vi "ColorPatternMatch_Setting_UI.vi"(0 "Vision_Image In":T3(plugin-control), 1 "Coord?":bool, 5 "List ROI 2":refnum<vi>, 7 "AlgIn":T2, 9 "ProjectName":string="CDF", 11 "error in (no error)":errorcluster, 12 "Parameter":string, 14 "RootPath":path) -> (4 "Analysis_Setting":string, 10 "Cancel?":bool, 15 "error out":errorcluster)   [LabVIEW 2019]
uses:
  Controls/V_Analysis_Type.ctl
  Controls/_UI Command Cluster/ColorMatch_UI Command.ctl
  <vilib>/Utility/miscctls.llb/LVPointTypeDef.ctl
  Controls/Analysis_Setting.ctl
  Controls/Color Pattern Match/Analysis Color Pattern Match Parameter.ctl
  <vilib>/vision/Image Controls.llb/IMAQ Image.ctl
  0394f2f0-e91b-465b-bb19-2289d360cfca.vi
  c15c5890-f854-46a2-b98b-929fa5ff6ec0.vi
  cb7ab341-9881-4345-8d5f-fb9cb1b2a84f.vi
  73ae4806-8b8b-4118-bada-9954a96a792c.vi
  76c2e7b3-0f24-4336-b544-f46512082401.vi
  <vilib>/JDP Science/JSONtext/JSON text to Variant.vi
  <vilib>/JDP Science/JSONtext/Variant to JSON Text.vi
  <vilib>/vision/NI_Vision_Development_Module.lvlib
  <vilib>/userdefined/High Color/IMAQdx.ctl
panel:
  out "ListROI":T1
  out "Bounding Box":cluster{"x":sgl, "y":sgl}[][](array[cluster])
  out "AlgOut":T2
  in  "Match Saturation Threshold":i32=80 min=10 max=255 step=1
  out "RunROI":T1
  in  "SetROI":bool
  out "TemplateROI":T1
  out "Template Image":T3(plugin-control)
  in  "Cancel":bool
  in  "Done":bool
  in  "ColorMatchTab":T4(tab)
  in  "AngleRange+/-":dbl
  in  "Color Score Weight":i32=750 min=0 max=1000
  in  "Match Offset":cluster{"X":dbl, "Y":dbl}
  in  "Number of Matches to Find":i32
  in  "Search Strategy":u32(ring) items=["Conservative", "Balance", "Aggressive", "VeryAggressive"]
  in  "Minimum Match Score":i32=750 min=0 max=1000
  in  "Color Sensitivity":u32(ring) items=["Low", "Medium", "High"]
  in  "Sub-Pixel Accuracy":bool
  in  "Match Mode":enum16{"Shift Invariant", "Rotation Invariant"}(ring)
  in  "IgnoreBlack And White":T5(ring)
  in  "Match Saturation Threshold 2":i32=80 min=10 max=255 step=1
  in  "Result":T6(array[cluster])
  out "Number of Matches":i32
  in  "Vision_Image":T3(plugin-control)
  in  "Run Algorithm":bool
  in  "SetTemplate":bool
  # "Use Ctrl to Select multiple ROI"
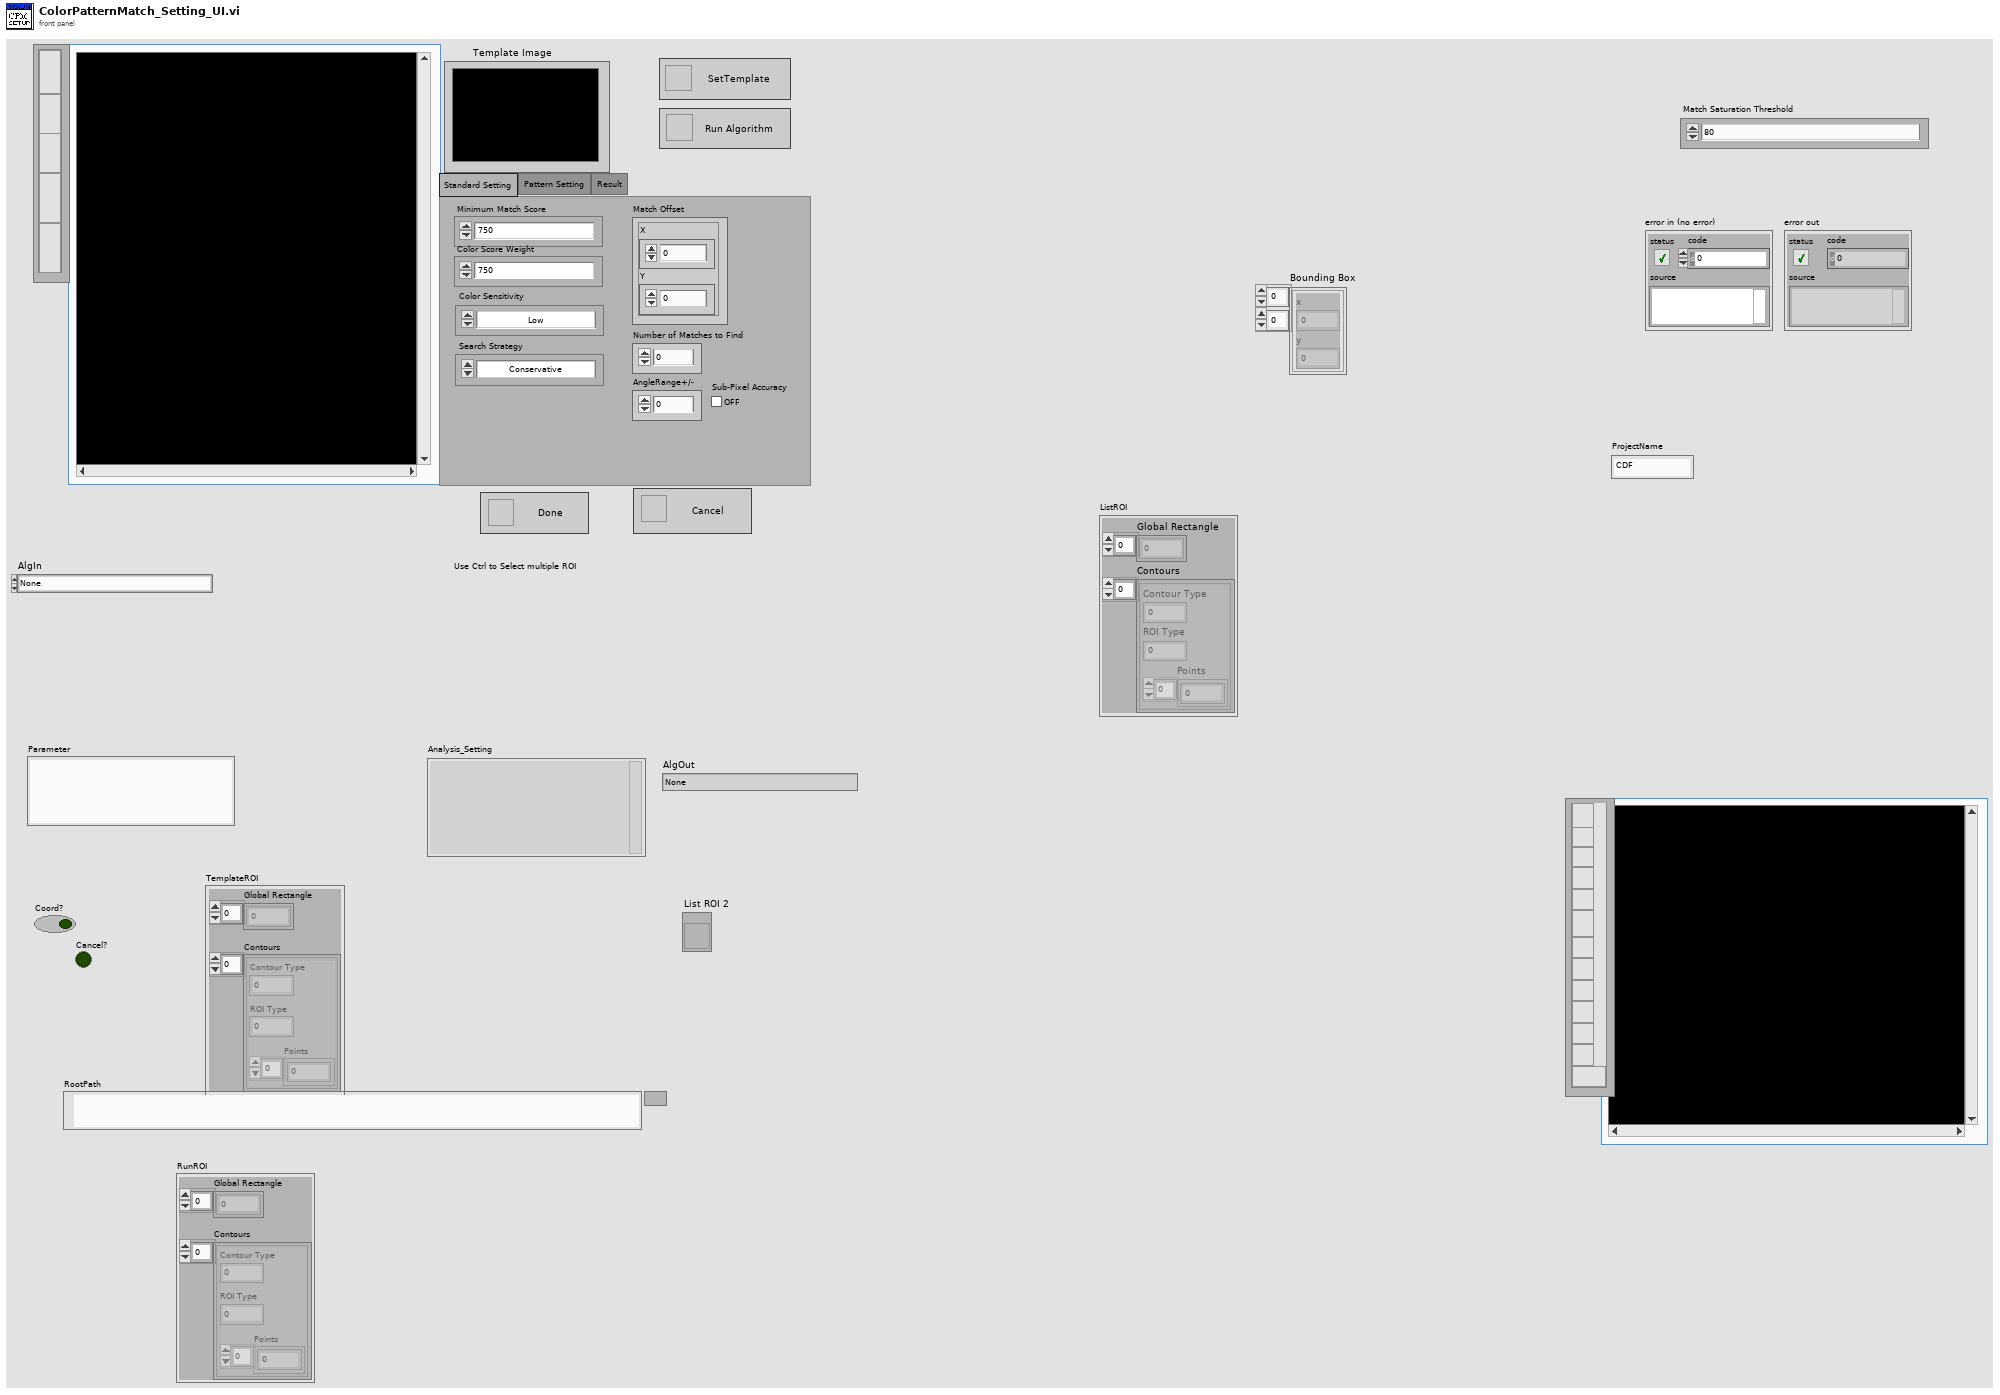
[diagram p1: front panel]
types:
  T1 = cluster{"Global Rectangle":i32[], "Contours":cluster{"Contour Type":u32, "ROI Type":u32, "Points":i32[]}[]}
  T2 = typedef "V_Analysis_Type.ctl" = enum16{"None", "C_Color Pattern Matching", "G_PatternMatching", "G_ShapeDectect", "G_GeometricMatch", "B_Area Check"}
  T3 = typedef "IMAQ Image.ctl" = refnum<image>
  T4 = enum32{"Standard Setting", "Pattern Setting", "Result"}
  T5 = enum16{"Disable", "IgnoreBlack", "IgnoreWhite", "IgnoreBlack And White"}
  T6 = cluster{"X":dbl, "Y":dbl, "Angle":dbl, "Score":dbl}[]
  T7 = typedef "Image Type" = u32
  T8 = typedef "ColorMatch_UI Command.ctl" = enum16{"Init", "Done", "Cancel", "RunAlgorithm", "SetTemplate", "SetROI", "ClearOverlay", "Load Template", "Draw Overlay", "Offset"}
  T9 = typedef "LVPointTypeDef.ctl" = cluster{"Horizontal":i16, "Vertical":i16}
  T10 = typedef "IMAQdx.ctl" = refnum<k21>
  T11 = typedef "Analysis_Setting.ctl" = cluster{"PreProcess":T2, "Parameter":string}
  T12 = enum8{"Enabled", "Disabled", "Disabled and Grayed Out"}
  T13 = typedef "Analysis Color Pattern Match Parameter.ctl" = cluster{"IgnoreBlack And White":enum16{"Disable", "IgnoreBlack", "IgnoreWhite", "IgnoreBlack And White"}, "Match Saturation Threshold":i32, "Minimum Match Score":i32, "Color Score Weight":i32, "Color Sensitivity":u32, "Search Strategy":u32, "Match Offset":cluster{"X":dbl, "Y":dbl}, "Number of Matches to Find":i32, "AngleRange+/-":dbl, "Sub-Pixel Accuracy":bool, "ROI Descriptor":T14, "TemplatePath":string, "Match Mode":enum16{"Shift Invariant", "Rotation Invariant"}}
  T14 = typedef "ROI Descriptor" = cluster{"Global Rectangle":i32[], "Contours":cluster{"ID":enum32{"External", "Internal"}, "Type":u32, "Coordinates":i32[]}[]}
  T15 = cluster{"Desired Font (Application)":enum16{"User-specified Font", "Application Font", "System Font", "Dialog Font"}, "[User-specified Font]":cluster{"Font Name":string, "Size":i16, "Strikeout?":bool, "Italic?":bool, "Underline?":bool, "Outline?":bool, "Shadow?":bool, "Bold?":bool, "Rotation Angle":dbl}, "Horizontal Alignment":i16, "Vertical Alignment":i16}
  T16 = cluster{"Contour Type":u32, "ROI Type":u32, "Points":i32[]}
  T17 = cluster{"Position":cluster{"x":sgl, "y":sgl}, "Angle":sgl, "Scale":sgl, "Score":sgl, "Bounding Box":cluster{"x":sgl, "y":sgl}[]}[]
  T18 = cluster{"x":sgl, "y":sgl, "Angle":sgl, "Score":sgl}
  T19 = cluster{"Contour Type":u32, "ROI Type":u32, "Points":i32[]}[]
  T20 = enum16{"Init", "Done", "Cancel", "RunAlgorithm", "SetTemplate", "SetROI", "ClearOverlay"}
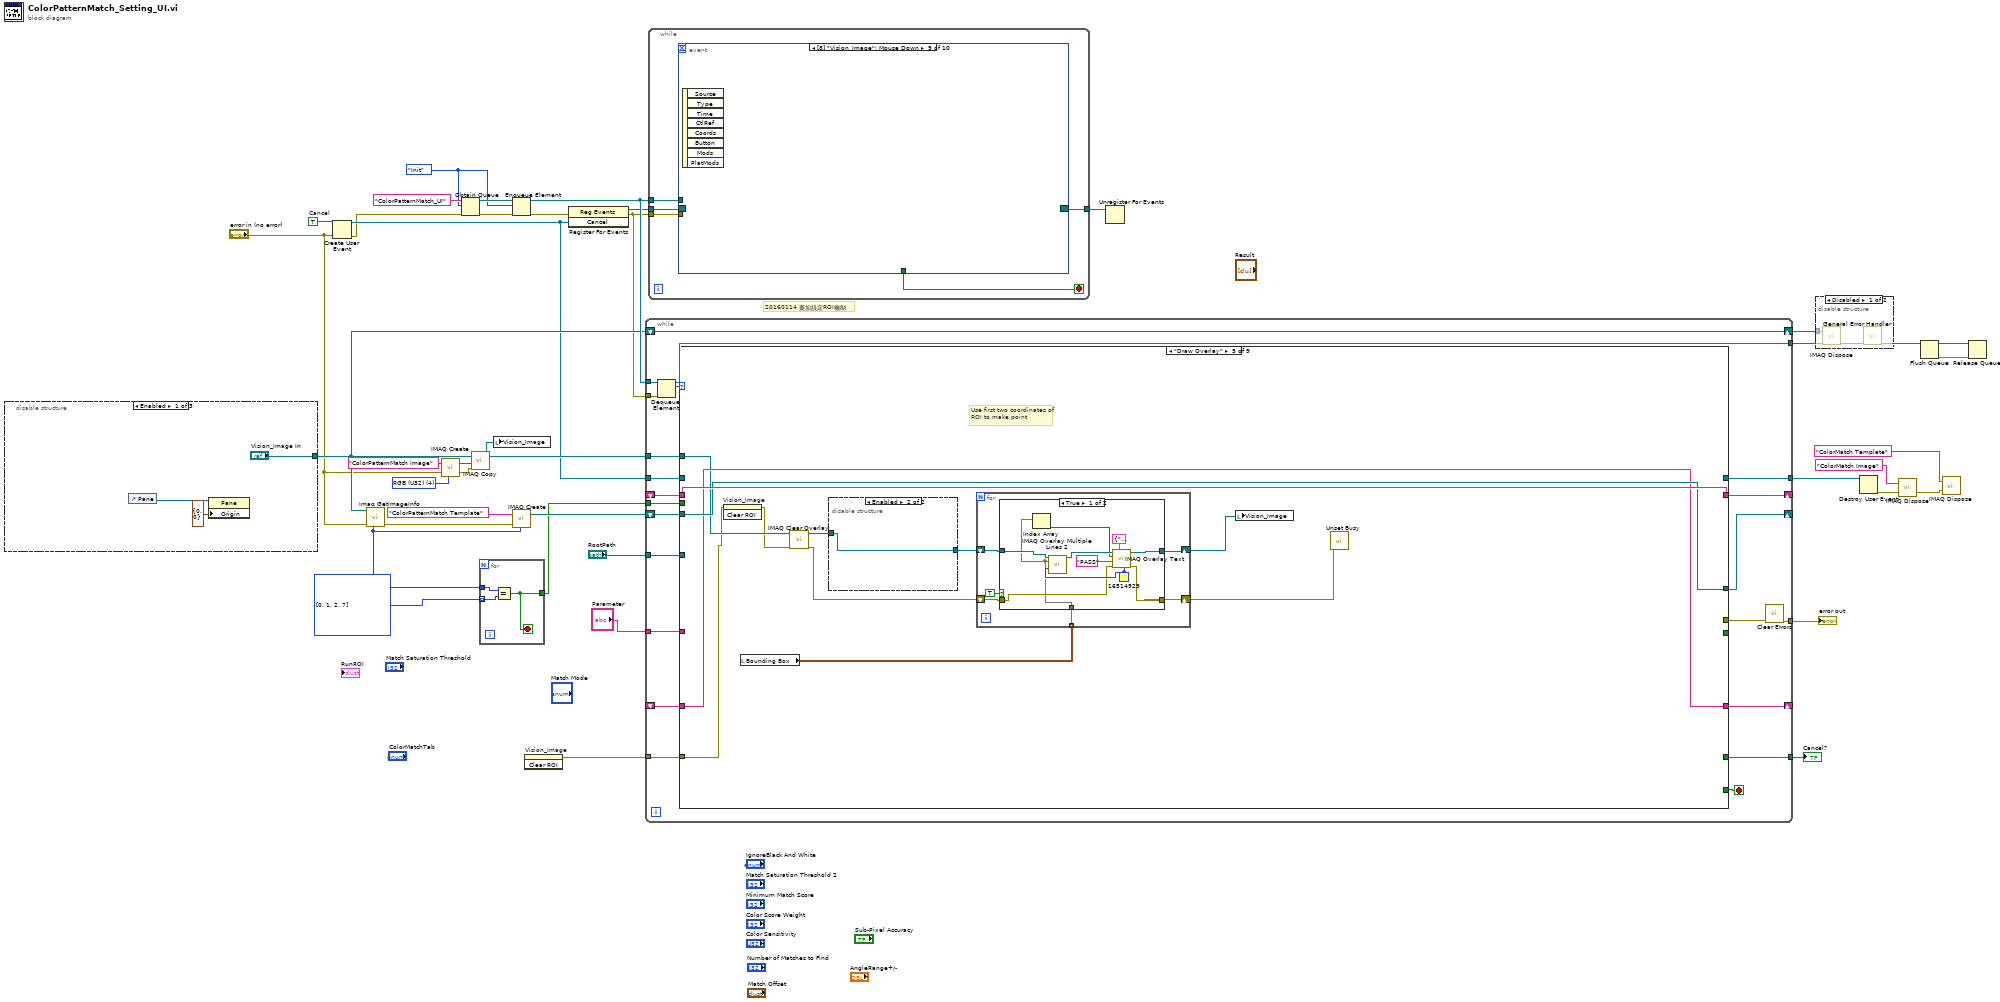
[diagram p0: block diagram]
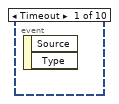
[diagram p2: hidden frame]
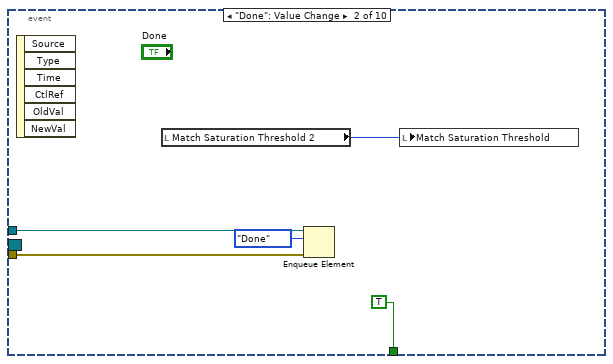
[diagram p3: hidden frame]
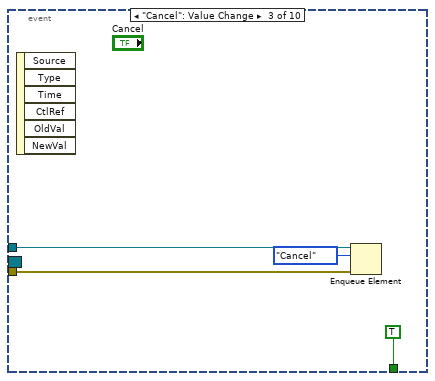
[diagram p4: hidden frame]
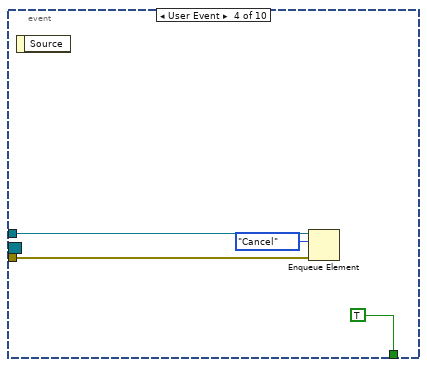
[diagram p5: hidden frame]
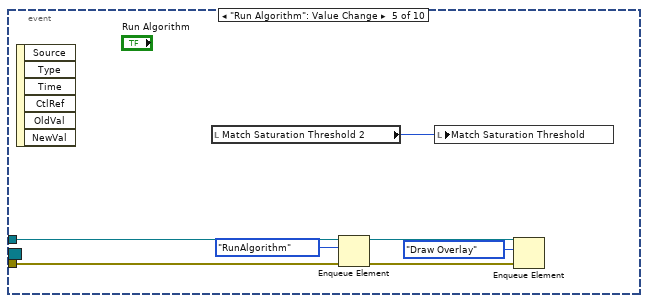
[diagram p6: hidden frame]
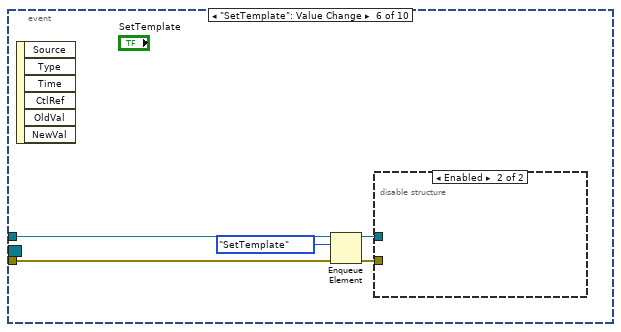
[diagram p7: hidden frame]
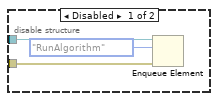
[diagram p8: hidden frame]
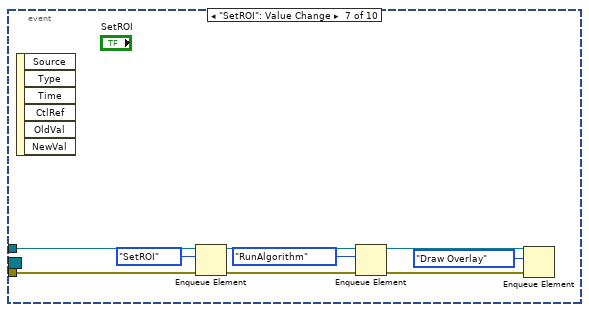
[diagram p9: hidden frame]
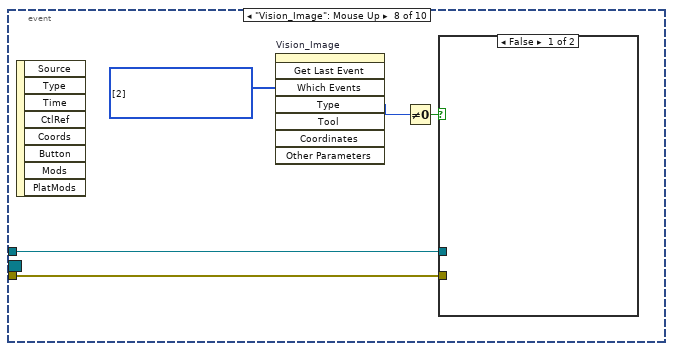
[diagram p10: hidden frame]
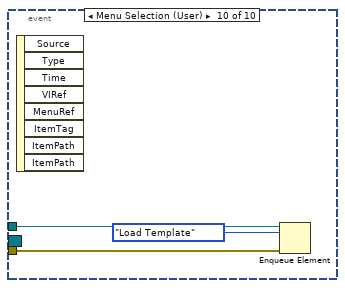
[diagram p12: hidden frame]
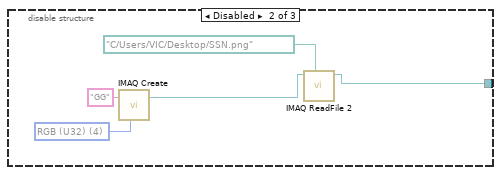
[diagram p13: hidden frame]
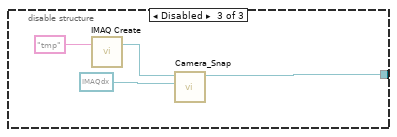
[diagram p14: hidden frame]
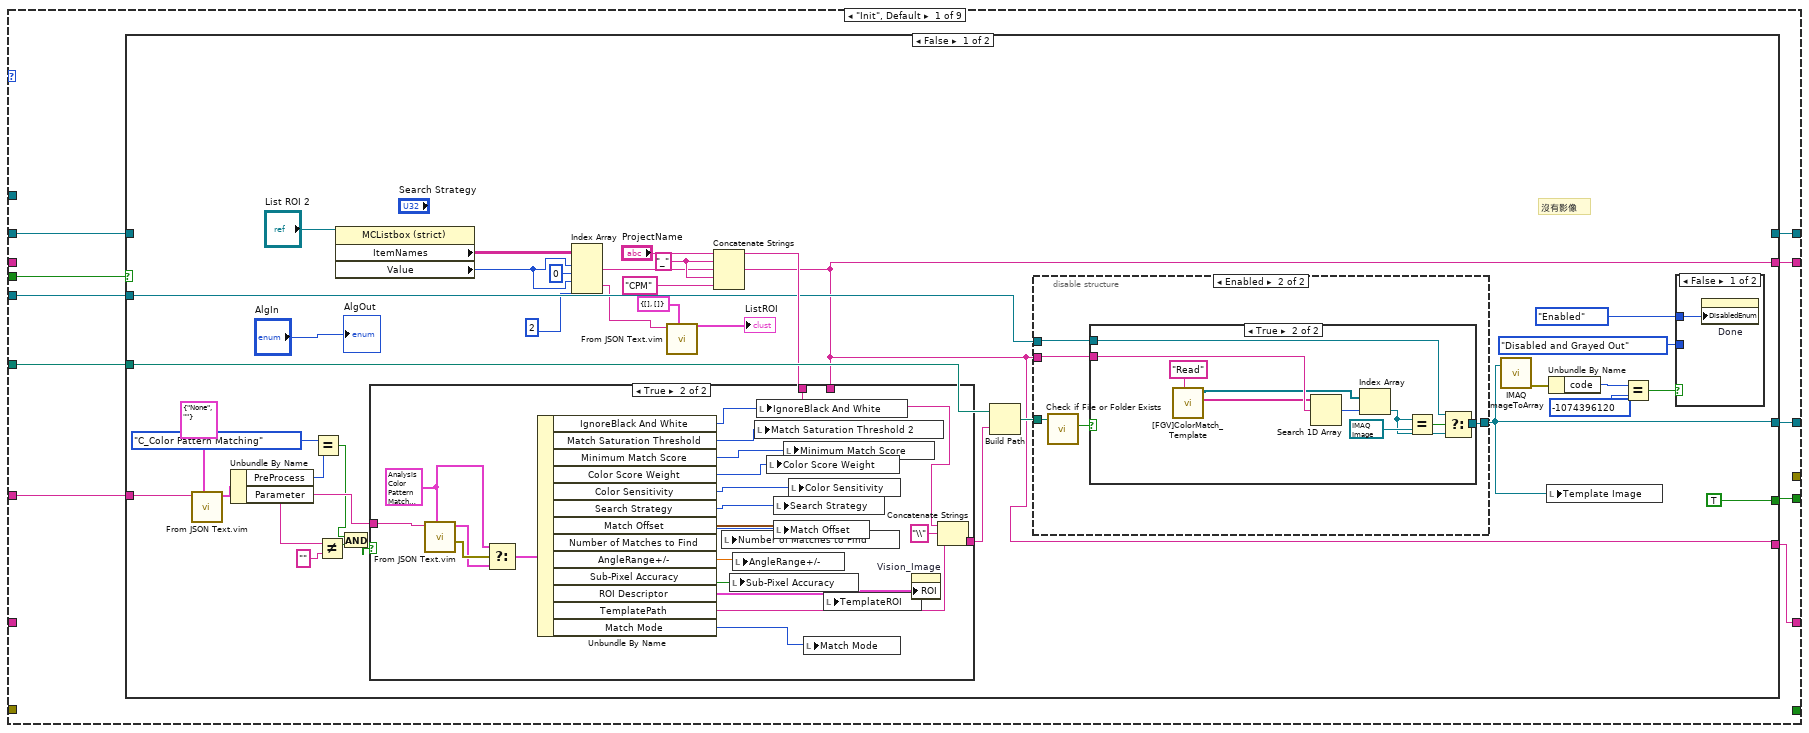
[diagram p16: hidden frame]
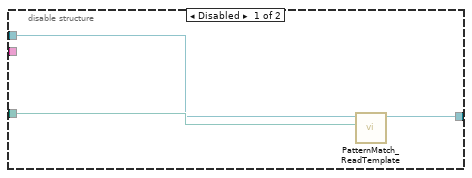
[diagram p17: hidden frame]
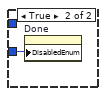
[diagram p19: hidden frame]
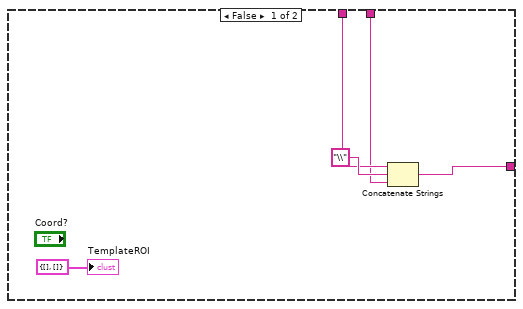
[diagram p20: hidden frame]
diagram:
  w2 = T7 4 items=["Grayscale (U8)", "Grayscale (I16)", "Grayscale (SGL)", "Complex (CSG)", "RGB (U32)", "HSL (U32)", "RGB (U64)", "Grayscale (U16)"] ("Image Type")
  w21 = TRUE  # Cancel
  w5 = T7[] [0, 1, 2, 7] items=["Grayscale (U8)", "Grayscale (I16)", "Grayscale (SGL)", "Complex (CSG)", "RGB (U32)", "HSL (U32)", "RGB (U64)", "Grayscale (U16)"] ("x")
  w22 = ColorMatch_UI_Command."Init"
  # "20160114 要加設定ROI機制"
  n1 = disable-structure shown="Enabled" {
    disable-tunnel: ["Vision_Image In" w44 w48] -> w25
    frame Enabled {
      n2 = control-ref of="Pane"() -> (w41:refnum<vi>)
      n3 = property class="Pane"(reference=w41, "Origin"=T9 {"Horizontal"=0, "Vertical"=0}) -> ()  [unwired: 1 in, 2 out]
    }
    frame Disabled {
      w47 = T7 4 items=["Grayscale (U8)", "Grayscale (I16)", "Grayscale (SGL)", "Complex (CSG)", "RGB (U32)", "HSL (U32)", "RGB (U64)", "Grayscale (U16)"] ("Image Type")
      n4 = call "IMAQ Create"("Image Name"="GG", "Image Type"=w47) -> ("New Image"=w45:T3)  [unwired: 3 in, 1 out]
      n5 = call "IMAQ ReadFile 2"("File Path"=path "C:/Users/VIC/Desktop/SSN.png", "Image"=w45) -> ("Image Out"=w44:T3)  [unwired: 5 in, 4 out]
    }
    frame Disabled {
      n6 = call "IMAQ Create"("Image Name"="tmp") -> ("New Image"=w49:T3)  [unwired: 4 in, 1 out]
      n7 = call "Camera_Snap.vi"("Camera Session In"=T10 refnum, "Image In"=w49) -> ("New Image"=w48:T3)  [unwired: 8 in, 1 out]
    }
  }
  n8 = Create User Event(user event datatype=w21, error in="error in (no error)") -> (user event=w19:refnum<user-event>, error out=w10:errorcluster)
  n9 = call "Imaq GetImageInfo"("error in (no error)"="error in (no error)", "Image"=w25) -> ("error out"=w8:errorcluster, "Image Type"=w6:T7)  [unwired: 2 in, 6 out]
  n10 = call "IMAQ Create"("Image Name"="ColorPatternMatch Image", "Image Type"=w2, "error in (no error)"="error in (no error)") -> ("New Image"=w34:T3, "error out"=w9:errorcluster)  [unwired: 2 in]
  n11 = Obtain Queue(name (unnamed)="ColorPatternMatch_UI", element data type=w22, error in (no error)=w10) -> (queue out=w31:refnum<queue>, error out=w30:errorcluster)  [unwired: 2 in, 1 out]
  n12 = call "IMAQ Copy"("error in (no error)"=w9, "Image Dst"=w34, "Image Src"=w25) -> ("Image Dst Out"=w33:T3)  [unwired: 3 in, 1 out]
  n13 = for {
    tunnel: w6 -> [w54]
    tunnel: w5 -> [w53] mode=indexing
    tunnel: [w52] -> w4
    stop <- w52 stop-if-true
    n14 = Equal?(x=w54, y=w53) -> (x = y?=w52:bool)
  }
  n15 = local write "Vision_Image"(w33) -> ()
  n16 = Enqueue Element(queue=w31, element=w22, error in (no error)=w30) -> (queue out=w27:refnum<queue>, error out=w16:errorcluster)  [unwired: 1 in, 1 out]
  n17 = call "IMAQ Create"("Image Name"="ColorPatternMatch Template", "Image Type"=w6, "error in (no error)"=w8) -> ("New Image"=w24:T3)  [unwired: 2 in, 1 out]
  n18 = invoke on="Vision_Image" class="ImageControl" method="Clear ROI"() -> (error out=w36:errorcluster)  [unwired: 3 in, 2 out]
  n19 = register-events(error in=w16, w19) -> (reference out=w20:refnum<event-registration>, error out=w15:errorcluster)  [unwired: 1 in]
  n20 = while {
    shift-right: [w76] -> w39
    shift-left: w25 -> [w76]
    tunnel: [w72] -> w38
    tunnel: w36 -> [w58]
    tunnel: w33 -> [w75]
    tunnel: w27 -> [w70]
    tunnel: w15 -> [w68]
    tunnel: [w67] -> w26
    shift-right: [w66] -> _
    shift-left: _ -> [w65]
    shift-right: [w63] -> _
    shift-left: w24 -> [w74]
    shift-right: [w64] -> _
    shift-left: _ -> [w73]
    tunnel: "RootPath" -> [w62]
    tunnel: w4 -> [w61]
    tunnel: w19 -> [w60]
    tunnel: [w59] -> w18
    tunnel: [w57] -> w3
    tunnel: "Parameter" -> [w55]
    stop <- w71 stop-if-true
    n21 = Dequeue Element(queue=w70, error in (no error)=w68) -> (queue out=w67:refnum<queue>, element=w69:T8)  [unwired: 1 in, 2 out]
    n22 = case shown="\"Draw Overlay\"" w69 {
      tunnel: [_ TRUE w207 _ _ _ _ _ _] -> w71
      tunnel: w75 -> [_ w199 w206 _ w283 _ _ _ _]
      tunnel: w74 -> [w81 _ w205 w211 w285 w325 w398 w408 w422]
      tunnel: [_ _ w207 _ _ _ _ _ _] -> w72
      tunnel: w73 -> [_ w187 w203 w209 w284 w326 w399 w409 w423]
      tunnel: [w85 w198 w204 w216 w286 w327 w400 w410 w424] -> w66
      tunnel: w65 -> [_ w198 w204 w216 w286 w327 w400 w410 w424]
      tunnel: [w83 w187 w203 w209 w284 w326 w399 w409 w423] -> w64
      tunnel: [w86 T3 refnum ("Template Out") T3 refnum ("Template Out") w211 w285 w322 w398 w408 w414] -> w63
      tunnel: [w84 FALSE _ _ _ w324 _ _ _] -> _
      tunnel: w62 -> [w82 _ _ _ _ w323 _ _ w421]
      tunnel: w61 -> [w80 _ _ _ _ _ _ _ _]
      tunnel: w60 -> [w79 w195 w201 _ _ _ _ _ _]
      tunnel: [w78 w195 w201 _ _ _ _ _ _] -> w59
      tunnel: w58 -> [_ _ _ _ w277 _ _ _ _]
      tunnel: [_ _ _ w208 _ _ _ _ _] -> w56
      tunnel: w55 -> [w77 _ _ _ _ _ _ _ _]
      frame "Init", Default {
        n23 = case shown="False" w80 {
          tunnel: [w114 _] -> w86
          tunnel: [w87 _] -> w85
          tunnel: [TRUE _] -> w84
          tunnel: [w87 _] -> w83
          tunnel: w82 -> [w121 _]
          tunnel: w81 -> [w115 _]
          tunnel: w79 -> [_ w172]
          tunnel: [_ w170] -> w78
          tunnel: w77 -> [w94 _]
          frame False {
            w118 = "_" ("string")
            # "沒有影像"
            n24 = call "From JSON Text.vim"("Data Type and Default Value"=T11 {"PreProcess"=enum."None", "Parameter"=""} ("Analysis_Setting In"), "JSON"=w94) -> ("Data out"=w102:T11)  [unwired: 8 in, 1 out]
            n25 = Unbundle By Name(w102) -> ("PreProcess"=w91:T2, "Parameter"=w101:string)
            n26 = Equal?(x=V_Analysis_Type."C_Color Pattern Matching", y=w91) -> (x = y?=w89:bool)
            n27 = Not Equal?(x=w101, y="") -> (x != y?=w93:bool)
            n28 = property class="MCListbox (strict)"(reference="List ROI 2") -> ("ItemNames"=w117:string[][], "Value"=w99:i32)  [unwired: 1 in, 2 out]
            n29 = And(x=w89, y=w93) -> (x .and. y?=w92:bool)
            n30 = Index Array(array=w117, index (row) #1=w99, index (col) #1=0 ("disabled index (col)"), index (row) #2=w99, index (col) #2=2 ("disabled index (col)")) -> (element #1=w104:string, element #2=w97:string)
            n31 = call "From JSON Text.vim"("Data Type and Default Value"=T1 {"Global Rectangle"=[], "Contours"=[]} ("ROI"), "JSON"=w97) -> ("Data out"=→"ListROI":T1)  [unwired: 8 in, 1 out]
            n32 = Concatenate Strings("ProjectName", w118, w104, w118, "CPM" ("string")) -> (w87:string)
            n33 = case shown="True" w92 {
              tunnel: [w144 w151] -> w88
              tunnel: "ProjectName" -> [w146 w150]
              tunnel: w101 -> [_ w169]
              tunnel: w87 -> [w145 _]
              frame False {
                n34 = Concatenate Strings(w146, "\\" ("string"), w145) -> (w144:string)
                "TemplateROI" <- T1 {"Global Rectangle"=[], "Contours"=[]} ("ROI")
              }
              frame True {
                w165 = T13 {"IgnoreBlack And White"=enum."IgnoreBlack And White", "Match Saturation Threshold"=80, "Minimum Match Score"=750, "Color Score Weight"=750, "Color Sensitivity"=1, "Search Strategy"=0, "Match Offset"={"X"=0.0, "Y"=0.0}, "Number of Matches to Find"=1, "AngleRange+/-"=0.0, "Sub-Pixel Accuracy"=FALSE, "ROI Descriptor"={"Global Rectangle"=[], "Contours"=[]}, "TemplatePath"="", "Match Mode"=enum."Shift Invariant"} ("Color Pattern Match")
                n35 = call "From JSON Text.vim"("Data Type and Default Value"=w165, "JSON"=w169) -> ("error out"=w168:errorcluster, "Data out"=w166:T13)  [unwired: 8 in]
                n36 = Select(t=w165, s=w168, f=w166) -> (s? t:f=w167:T13)
                n37 = Unbundle By Name(w167) -> ("IgnoreBlack And White"=w154:T5, "Match Saturation Threshold"=w153:i32, "Minimum Match Score"=w156:i32, "Color Score Weight"=w155:i32, "Color Sensitivity"=w163:u32, "Search Strategy"=w162:u32, "Match Offset"=w161:cluster{"X":dbl, "Y":dbl}, "Number of Matches to Find"=w160:i32, "AngleRange+/-"=w159:dbl, "Sub-Pixel Accuracy"=w158:bool, "ROI Descriptor"=w164:T14, "TemplatePath"=w157:string, "Match Mode"=w152:enum16{"Shift Invariant", "Rotation Invariant"})
                n38 = local write "Number of Matches to Find"(w160) -> ()
                n39 = local write "Sub-Pixel Accuracy"(w158) -> ()
                n40 = local write "AngleRange+/-"(w159) -> ()
                n41 = local write "Match Saturation Threshold 2"(w153) -> ()
                n42 = local write "IgnoreBlack And White"(w154) -> ()
                n43 = local write "Color Score Weight"(w155) -> ()
                n44 = local write "Search Strategy"(w162) -> ()
                n45 = local write "Match Offset"(w161) -> ()
                n46 = local write "Minimum Match Score"(w156) -> ()
                n47 = local write "Color Sensitivity"(w163) -> ()
                n48 = local write "Match Mode"(w152) -> ()
                n49 = local write "TemplateROI"(w164) -> ()
                n50 = property on="Vision_Image" class="ImageControl"("ROI"=w164) -> ()  [unwired: 2 in, 2 out]
                n51 = Concatenate Strings(w150, "\\" ("string"), w157) -> (w151:string)
              }
            }
            n52 = Build Path(base path=w121, name or relative path=w88) -> (appended path=w116:path)
            n53 = disable-structure shown="Enabled" {
              disable-tunnel: w116 -> [w125 w129]
              disable-tunnel: w115 -> [w124 w126]
              disable-tunnel: [w123 w127] -> w114
              disable-tunnel: w87 -> [_ w130]
              frame Disabled {
                n54 = call "PatternMatch_ReadTemplate.vi"("template path"=w125, "Template"=w124) -> ("Template Out"=w123:T3)  [unwired: 8 in, 1 out]
              }
              frame Enabled {
                n55 = call <vilib>:"Check if File or Folder Exists.vi"("path"=w129) -> ("file or folder exists?"=w128:bool)  [unwired: 8 in, 2 out]
                n56 = case shown="True" w128 {
                  tunnel: w130 -> [_ w141]
                  tunnel: [w131 w135] -> w127
                  tunnel: w126 -> [w131 w137]
                  frame False {
                  }
                  frame True {
                    n57 = call "[FGV]ColorMatch_Template.vi"("CMTemplateCommand"="Read") -> ("Image Name Array 2"=w132:string[], "Image Array 2"=w133:T3[])  [unwired: 8 in, 1 out]
                    n58 = Search 1D Array(1D array=w132, element=w141) -> (index of element=w140:i32)  [unwired: 1 in]
                    n59 = Index Array(array=w133, index=w140) -> (element=w136:T3)
                    n60 = Equal?(x=w136, y=T3 refnum) -> (x = y?=w138:bool)
                    n61 = Select(t=w137, s=w138, f=w136) -> (s? t:f=w135:T3)
                  }
                }
              }
            }
            n62 = call "IMAQ ImageToArray"("Image"=w114) -> ("error out"=w111:errorcluster)  [unwired: 3 in, 4 out]
            n63 = local write "Template Image"(w114) -> ()
            n64 = Unbundle By Name(w111) -> ("code"=w110:i32)
            n65 = Equal?(x=w110, y=-1074396120) -> (x = y?=w108:bool)
            n66 = case shown="False" w108 {
              tunnel: T12."Disabled and Grayed Out" ("Disabled") -> [_ w143]
              tunnel: T12."Enabled" ("Disabled") -> [w142 _]
              frame False {
                n67 = property on="Done" class="Bool"("DisabledEnum"=w142) -> ()  [unwired: 2 in, 2 out]
              }
              frame True {
                n68 = property on="Done" class="Bool"("DisabledEnum"=w143) -> ()  [unwired: 2 in, 2 out]
              }
            }
            "AlgOut" <- "AlgIn"
          }
          frame True {
            # "輸入進來若是RGB則關閉"
            n69 = One Button Dialog(message="The Input Image Error,Image Grayscale", button name ("OK")="Cancel") -> (true=w171:bool)
            n70 = Generate User Event(user event=w172, event data cluster=w171) -> (user event out=w170:refnum<user-event>)  [unwired: 2 in, 1 out]
          }
        }
      }
      frame "Done" {
        w193 = T11 {"PreProcess"=enum."None", "Parameter"=""}  # Analysis_Setting
        (unwired) T16 {"Contour Type"=0, "ROI Type"=0, "Points"=[]} ("RegionContour")
        n71 = local read "Color Score Weight"() -> (w180:i32)
        n72 = local read "Minimum Match Score"() -> (w179:i32)
        n73 = local read "Match Saturation Threshold 2"() -> (w177:i32)
        n74 = call "IMAQ Dispose"("Image"=w199) -> ()  [unwired: 5 in, 1 out]
        n75 = local read "Sub-Pixel Accuracy"() -> (w186:bool)
        n76 = local read "Number of Matches to Find"() -> (w184:i32)
        n77 = local read "IgnoreBlack And White"() -> (w178:T5)
        n78 = local read "AngleRange+/-"() -> (w185:dbl)
        n79 = local read "Search Strategy"() -> (w182:u32)
        n80 = local read "Match Offset"() -> (w183:cluster{"X":dbl, "Y":dbl})
        n81 = local read "Color Sensitivity"() -> (w181:u32)
        n82 = local read "TemplateROI"() -> (w175:T1)
        n83 = property on="Vision_Image" class="ImageControl"("ROI"=w175) -> ()  [unwired: 2 in, 2 out]
        n84 = local read "Match Mode"() -> (w176:enum16{"Shift Invariant", "Rotation Invariant"})
        n85 = Bundle By Name(cluster=T13 {"IgnoreBlack And White"=enum."IgnoreBlack And White", "Match Saturation Threshold"=80, "Minimum Match Score"=750, "Color Score Weight"=750, "Color Sensitivity"=1, "Search Strategy"=0, "Match Offset"={"X"=0.0, "Y"=0.0}, "Number of Matches to Find"=1, "AngleRange+/-"=0.0, "Sub-Pixel Accuracy"=FALSE, "ROI Descriptor"={"Global Rectangle"=[], "Contours"=[]}, "TemplatePath"="", "Match Mode"=enum."Shift Invariant"} ("Color Pattern Match"), "IgnoreBlack And White"=w178, "Match Saturation Threshold"=w177, "Minimum Match Score"=w179, "Color Score Weight"=w180, "Color Sensitivity"=w181, "Search Strategy"=w182, "Match Offset"=w183, "Number of Matches to Find"=w184, "AngleRange+/-"=w185, "Sub-Pixel Accuracy"=w186, "ROI Descriptor"=w175, "TemplatePath"=w187, "Match Mode"=w176) -> (w194:T13)
        n86 = call "To JSON Text.vim"("Anything"=w194) -> ("<JSON>"=w192:string)  [unwired: 9 in, 1 out]
        n87 = local read "AlgOut"() -> (w189:T2)
        n88 = Bundle(cluster=w193, "PreProcess"=w189, "Parameter"=w192) -> (w191:T11)
        n89 = call "To JSON Text.vim"("Anything"=w191) -> ("<JSON>"=→"Analysis_Setting":string)  [unwired: 9 in, 1 out]
      }
      frame "Cancel" {
        w207 = TRUE
        n90 = call "IMAQ Dispose"("Image"=w205) -> ()  [unwired: 5 in, 1 out]
        n91 = call "IMAQ Dispose"("Image"=w206) -> ()  [unwired: 5 in, 1 out]
      }
      frame "RunAlgorithm" {
        n92 = call "Imaq GetImageInfo"("Image"=w211) -> ("Y Resolution"=w215:i32, "X Resolution"=w214:i32)  [unwired: 3 in, 6 out]
        n93 = Equal To 0?(x=w214) -> (x = 0?=w213:bool)
        n94 = Equal To 0?(x=w215) -> (x = 0?=w212:bool)
        n95 = Or(x=w213, y=w212) -> (x .or. y?=w210:bool)
        n96 = case shown="False" w210 {
          tunnel: w211 -> [w223 _]
          tunnel: w209 -> [w222 _]
          tunnel: [w221 _] -> w208
          frame False {
            n97 = local read "Vision_Image"() -> (w224:T3)
            n98 = property on="Vision_Image" class="ImageControl"() -> ("ROI"=w217:T1)  [unwired: 2 in, 2 out]
            n99 = call <vilib>:"Set Busy.vi"() -> ("error out"=w227:errorcluster)  [unwired: 10 in, 1 out]
            n100 = Unbundle(w217) -> ("Global Rectangle"=w219:i32[])  [unwired: 1 out]
            n101 = Empty Array?(array=w219) -> (empty?=w218:bool)
            n102 = call "IMAQ Clear Overlay"("error in (no error)"=w227, "Image"=w224) -> ("error out"=w225:errorcluster, "Image Out"=w226:T3)  [unwired: 8 in]
            n103 = case shown="True" w218 {
              tunnel: [w228 w229] -> w220
              tunnel: w217 -> [w228 _]
              frame False {
                n104 = local write "RunROI"(w228) -> ()
              }
              frame True {
                n105 = local read "RunROI"() -> (w229:T1)
              }
            }
            n106 = disable-structure shown="Enabled" {
              disable-tunnel: w223 -> [w239 _]
              disable-tunnel: w225 -> [w238 w264]
              disable-tunnel: _ -> [w236 _]
              disable-tunnel: _ -> [w235 _]
              disable-tunnel: _ -> [w234 _]
              disable-tunnel: w226 -> [w233 w265]
              disable-tunnel: w220 -> [w230 w243]
              disable-tunnel: w222 -> [_ w248]
              disable-tunnel: [_ w263] -> w221
              frame Disabled {
                w241 = 0 items=["All", "Low Discrepancy Sampling", "Grayscale Value Pyramid", "Gradients Pyramid"] ("Algorithm")
                n107 = call "IMAQ Learn Pattern 4"("Algorithm"=w241, "error in (no error)"=w238, "Angle Range"=cluster{"Start Angle":sgl, "End Angle":sgl} {"Start Angle"=0.0, "End Angle"=360.0}, "Image"=w239) -> ("error out"=w237:errorcluster, "Template Image Out"=w231:T3)  [unwired: 5 in, 1 out]
                n108 = call "IMAQ Match Pattern 4"("Image"=w233, "Algorithm"=w235, "Template Image"=w231, "ROI Descriptor"=w230, "Parameters"=w236, "error in (no error)"=w237, "Advanced Options"=w234) -> ("Matches (pixel)"=w232:T17)  [unwired: 4 in, 4 out]
              }
              frame Enabled {
                n109 = local read "Color Score Weight"() -> (w255:i32)
                n110 = property on="Vision_Image" class="ImageControl"("ROI"=w243) -> ()  [unwired: 2 in, 2 out]
                n111 = local read "Minimum Match Score"() -> (w254:i32)
                n112 = local read "Match Saturation Threshold 2"() -> (w252:i32)
                n113 = local read "Match Mode"() -> (w251:enum16{"Shift Invariant", "Rotation Invariant"})
                n114 = local read "Sub-Pixel Accuracy"() -> (w261:bool)
                n115 = local read "Number of Matches to Find"() -> (w259:i32)
                n116 = local read "IgnoreBlack And White"() -> (w253:T5)
                n117 = local read "AngleRange+/-"() -> (w260:dbl)
                n118 = local read "Search Strategy"() -> (w257:u32)
                n119 = local read "Match Offset"() -> (w258:cluster{"X":dbl, "Y":dbl})
                n120 = local read "Color Sensitivity"() -> (w256:u32)
                n121 = Bundle By Name(cluster=T13 {"IgnoreBlack And White"=enum."IgnoreBlack And White", "Match Saturation Threshold"=80, "Minimum Match Score"=750, "Color Score Weight"=750, "Color Sensitivity"=1, "Search Strategy"=0, "Match Offset"={"X"=0.0, "Y"=0.0}, "Number of Matches to Find"=1, "AngleRange+/-"=0.0, "Sub-Pixel Accuracy"=FALSE, "ROI Descriptor"={"Global Rectangle"=[], "Contours"=[]}, "TemplatePath"="", "Match Mode"=enum."Shift Invariant"} ("Color Pattern Match"), "IgnoreBlack And White"=w253, "Match Saturation Threshold"=w252, "Minimum Match Score"=w254, "Color Score Weight"=w255, "Color Sensitivity"=w256, "Search Strategy"=w257, "Match Offset"=w258, "Number of Matches to Find"=w259, "AngleRange+/-"=w260, "Sub-Pixel Accuracy"=w261, "ROI Descriptor"=w243, "TemplatePath"=w248, "Match Mode"=w251) -> (w249:T13)
                n122 = call "ColorPatternMatch_MainFunction.vi"("Image in"=w265, "Color Pattern Match"=w249, "ROI Descriptor"=T14 {"Global Rectangle"=[], "Contours"=[]}, "error in"=w264) -> ("Image Out"=w262:T3, "Matches out"=w246:T17, "Number of Matches"=→"Number of Matches":i32, "error out"=w263:errorcluster)  [unwired: 7 in, 1 out]
                n123 = for {
                  tunnel: w246 -> [w273] mode=indexing
                  tunnel: [w267] -> w245 mode=indexing
                  tunnel: [w266] -> w244 mode=indexing
                  n124 = Unbundle(w273) -> ("Position"=w272:cluster{"x":sgl, "y":sgl}, "Angle"=w269:sgl, "Score"=w268:sgl, "Bounding Box"=w266:cluster{"x":sgl, "y":sgl}[])  [unwired: 1 out]
                  n125 = Unbundle(w272) -> ("x"=w271:sgl, "y"=w270:sgl)
                  n126 = Bundle("x"=w271, "y"=w270, "Angle"=w269, "Score"=w268) -> (w267:T18)  [unwired: 1 in]
                }
                "Bounding Box" <- w244
                n127 = local write "Vision_Image"(w262) -> ()
                n128 = local write "Result"(w245) -> ()
              }
            }
          }
          frame True {
            n129 = One Button Dialog(message="No Template is Set~!!!\nPlease Set Template Before Analyze~!!") -> ()  [unwired: 1 in, 1 out]
          }
        }
      }
      frame "Draw Overlay" {
        # "Use first two coordinates of ROI to make point"
        n130 = invoke on="Vision_Image" class="ImageControl" method="Clear ROI"(error in=w277) -> (error out=w276:errorcluster)  [unwired: 2 in, 2 out]
        n131 = local read "Bounding Box"() -> (w275:cluster{"x":sgl, "y":sgl}[][])
        n132 = call "IMAQ Clear Overlay"("error in (no error)"=w276, "Image"=w283) -> ("error out"=w282:errorcluster, "Image Out"=w279:T3)  [unwired: 8 in]
        n133 = disable-structure shown="Enabled" {
          disable-tunnel: w279 -> [w290 w291]
          disable-tunnel: [w289 w291] -> w278
          frame Disabled {
            n134 = local read "ListROI"() -> (w287:T1)
            n135 = call "IMAQ Overlay ROI"("Colors (Green)"=u32[] [9567230], "ROI Descriptor"=w287, "Image"=w290) -> ("Image Out"=w289:T3)  [unwired: 7 in, 1 out]
          }
          frame Enabled {
          }
        }
        n136 = for {
          shift-right: [w295] -> w281
          shift-left: w282 -> [w296]
          shift-right: [w294] -> w280
          shift-left: w278 -> [w297]
          tunnel: w275 -> [w293] mode=indexing
          n137 = case shown="True" TRUE {
            tunnel: w297 -> [w303 w313]
            tunnel: w296 -> [w300 w310]
            tunnel: [w305 w315] -> w294
            tunnel: [w304 w314] -> w295
            tunnel: w293 -> [w299 w309]
            frame True {
              w302 = u32 16514929 ("BG Color (Transparent)")
              n138 = Index Array(array=w299) -> (element=w298:cluster{"x":sgl, "y":sgl})  [unwired: 1 in]
              n139 = call "IMAQ Overlay Multiple Lines 2"("Image"=w303, "Line End Points"=w299, "Color"=w302) -> ("Image Out"=w301:T3)  [unwired: 11 in, 1 out]
              n140 = call "IMAQ Overlay Text"("BG Color (Transparent)"=w302, "Font, Size & Style"=T15 {"Desired Font (Application)"=enum."Application Font", "[User-specified Font]"={"Font Name"="", "Size"=12, "Strikeout?"=FALSE, "Italic?"=FALSE, "Underline?"=FALSE, "Outline?"=FALSE, "Shadow?"=FALSE, "Bold?"=FALSE, "Rotation Angle"=0.0}, "Horizontal Alignment"=0, "Vertical Alignment"=1}, "error in (no error)"=w300, "String"="PASS", "Origin"=w298, "Image"=w301) -> ("error out"=w304:errorcluster, "Image Out"=w305:T3)  [unwired: 4 in]
            }
            frame False {
              w312 = u32 16711680 ("BG Color (Transparent)")
              n141 = Index Array(array=w309) -> (element=w308:cluster{"x":sgl, "y":sgl})  [unwired: 1 in]
              n142 = call "IMAQ Overlay Multiple Lines 2"("Image"=w313, "Line End Points"=w309, "Color"=w312) -> ("Image Out"=w311:T3)  [unwired: 11 in, 1 out]
              n143 = call "IMAQ Overlay Text"("BG Color (Transparent)"=w312, "Font, Size & Style"=T15 {"Desired Font (Application)"=enum."Application Font", "[User-specified Font]"={"Font Name"="", "Size"=12, "Strikeout?"=FALSE, "Italic?"=FALSE, "Underline?"=FALSE, "Outline?"=FALSE, "Shadow?"=FALSE, "Bold?"=FALSE, "Rotation Angle"=0.0}, "Horizontal Alignment"=0, "Vertical Alignment"=1}, "error in (no error)"=w310, "String"="NG", "Origin"=w308, "Image"=w311) -> ("error out"=w314:errorcluster, "Image Out"=w315:T3)  [unwired: 4 in]
            }
          }
        }
        n144 = local write "Vision_Image"(w280) -> ()
        n145 = call <vilib>:"Unset Busy.vi"("error in (no error)"=w281) -> ()  [unwired: 10 in, 1 out]
      }
      frame "SetTemplate" {
        # "沒有影像"
        # "-1074396120"
        n146 = call "Imaq GetImageInfo"("Image"=w325) -> ("error out"=w321:errorcluster)  [unwired: 3 in, 7 out]
        n147 = Unbundle By Name(w321) -> ("code"=w320:i32)
        n148 = Equal?(x=w320, y=-1074396120) -> (x = y?=w318:bool)
        n149 = case shown="True" w318 {
          tunnel: [w330 TRUE] -> w328
          frame False {
            n150 = Two Button Dialog(message="Template Already Exist, You Sure to Create New Template?") -> (T button?=w330:bool)  [unwired: 2 in]
          }
          frame True {
          }
        }
        n151 = case shown="True" w328 {
          tunnel: w325 -> [w332 w342]
          tunnel: w326 -> [_ w341]
          tunnel: [_ w340] -> w324
          tunnel: w323 -> [_ w339]
          tunnel: [w332 w338] -> w322
          frame False {
          }
          frame True {
            n152 = property on="Vision_Image" class="ImageControl"() -> ("ROI"=w337:T1)  [unwired: 2 in, 2 out]
            n153 = local read "Match Saturation Threshold 2"() -> (w333:i32)
            n154 = local read "IgnoreBlack And White"() -> (w334:T5)
            n155 = local read "AngleRange+/-"() -> (w335:dbl)
            n156 = local read "Sub-Pixel Accuracy"() -> (w336:bool)
            n157 = Unbundle By Name(w337) -> ("Contours"=w346:T19, "Global Rectangle"=w343:i32[])
            n158 = local write "TemplateROI"(w337) -> ()
            n159 = Array Size(array=w346) -> (size(s)=w345:i32)
            n160 = Not Equal To 0?(x=w345) -> (x != 0?=w344:bool)
            n161 = case shown="True" w344 {
              tunnel: w343 -> [_ w381]
              tunnel: w342 -> [w347 w380]
              tunnel: w341 -> [_ w352]
              tunnel: [_ TRUE] -> w340
              tunnel: w339 -> [_ w350]
              tunnel: [w347 w374] -> w338
              tunnel: w336 -> [_ _]
              tunnel: w335 -> [_ w369]
              tunnel: w334 -> [_ w364]
              tunnel: w333 -> [_ w363]
              frame False {
                n162 = One Button Dialog(message="Please Select Template On the Image") -> ()  [unwired: 1 in, 1 out]
              }
              frame True {
                w358 = T7 4 items=["Grayscale (U8)", "Grayscale (I16)", "Grayscale (SGL)", "Complex (CSG)", "RGB (U32)", "HSL (U32)", "RGB (U64)", "Grayscale (U16)"] ("Image Type")
                w365 = u32 0 items=["Color and Shape", "Color", "Shape "] ("Feature Mode")
                n163 = local read "ProjectName"() -> (w349:string)
                n164 = call <vilib>:"Set Busy.vi"() -> ("error out"=w375:errorcluster)  [unwired: 10 in, 1 out]
                n165 = local read "Match Mode"() -> (w367:enum16{"Shift Invariant", "Rotation Invariant"})
                n166 = Build Path(base path=w350, name or relative path=w349) -> (appended path=w351:path)
                n167 = Negate(x=w369) -> (-x=w370:dbl)
                n168 = Bundle(cluster=cluster{sgl, sgl} {0.0, 0.0}, w370, w369) -> (w368:cluster{sgl, sgl})
                n169 = Build Path(base path=w351, name or relative path=w352) -> (appended path=w377:path)
                n170 = call "[FGV]ColorMatch_Template.vi"("CMTemplateCommand"="Read") -> ("Image Name Array 2"=w353:string[])  [unwired: 8 in, 2 out]
                n171 = Build Array(w368) -> ()  [unwired: 1 out]
                n172 = call "IMAQ Extract"("Optional Rectangle"=w381, "error in (no error)"=w375, "Image Dst"=w380, "Image Src"="Vision_Image") -> ("error out"=w376:errorcluster, "Image Dst Out"=w372:T3)  [unwired: 6 in]
                n173 = case shown="\"Rotation Invariant\"" w367 {
                  tunnel: [w386 w387] -> w366
                  frame "Shift Invariant", Default {
                    w386 = u32 1 items=["All", "Shift Information", "Rotation Information"] ("Learn Mode")
                  }
                  frame "Rotation Invariant" {
                    w387 = u32 2 items=["All", "Shift Information", "Rotation Information"] ("Learn Mode")
                  }
                }
                n174 = Search 1D Array(1D array=w353, element=w352) -> (index of element=w355:i32)  [unwired: 1 in]
                n175 = Less Than 0?(x=w355) -> (x < 0?=w354:bool)
                n176 = case shown="True" w354 {
                  tunnel: w353 -> [_ w384]
                  tunnel: w352 -> [_ w383]
                  frame False {
                  }
                  frame True {
                    n177 = Build Array (concatenate)(w384, w383) -> (w382:string[])
                    n178 = call "[FGV]ColorMatch_Template.vi"("CMTemplateCommand"="Save", "Image Name Array"=w382, "Image Array"=w382) -> ()  [unwired: 6 in, 3 out]
                  }
                }
                n179 = invoke on="Vision_Image" class="ImageControl" method="Clear ROI"(error in=w376) -> ()  [unwired: 2 in, 3 out]
                n180 = call "IMAQ Setup Learn Color Pattern"("Saturation Threshold"=w363, "Ignore Black and White"=w364, "Feature Mode"=w365, "Learn Mode"=w366) -> ("error out"=w360:errorcluster, "Learn Color Pattern Setup Data"=w362:string)  [unwired: 6 in]
                n181 = call "IMAQ Create"("Image Name"=w352, "Image Type"=w358) -> ("New Image"=w357:T3)  [unwired: 3 in, 1 out]
                n182 = call "IMAQ Learn Color Pattern"("error in (no error)"=w360, "Learn Color Pattern Setup Data"=w362, "Image"=w372) -> ("error out"=w359:errorcluster, "Template Image Out"=w361:T3)  [unwired: 7 in]
                n183 = case shown="No Error" w359 {
                  tunnel: w377 -> [w394 _]
                  tunnel: w361 -> [w391 _]
                  tunnel: [w388 T3 refnum ("Image Dst Out")] -> w374
                  tunnel: [w392 _] -> w373
                  tunnel: w357 -> [w389 _]
                  frame No Error {
                    n184 = property on="Done" class="Bool"("DisabledEnum"=T12."Enabled" ("Disabled")) -> ()  [unwired: 2 in, 2 out]
                    n185 = call-poly "IMAQ Write File 2"("File Path"=w394, "Image"=w391) -> ("error out"=w392:errorcluster, "Image Out (duplicate)"=w390:T3)  [unwired: 8 in]
                    n186 = call "IMAQ Copy"("Image Dst"=w389, "Image Src"=w390) -> ("Image Dst Out"=w388:T3)  [unwired: 4 in, 1 out]
                  }
                  frame Error {
                    n187 = One Button Dialog(message="Invalid learn setup data.\nplease Reset Set", button name ("OK")="OK") -> ()  [unwired: 1 out]
                  }
                }
                "Template Image" <- w374
                n188 = call <vilib>:"Unset Busy.vi"("error in (no error)"=w373) -> ()  [unwired: 10 in, 1 out]
              }
            }
          }
        }
      }
      frame "SetROI" {
        n189 = property on="Vision_Image" class="ImageControl"() -> ("ROI"=w401:T1)  [unwired: 2 in, 2 out]
        n190 = Unbundle By Name(w401) -> ("Global Rectangle"=w403:i32[])
        n191 = Array Size(array=w403) -> (size(s)=w404:i32)
        n192 = Not Equal To 0?(x=w404) -> (x != 0?=w402:bool)
        n193 = case shown="True" w402 {
          tunnel: w401 -> [_ w406]
          frame False {
            n194 = One Button Dialog(message="Please Select An Area As ROI") -> ()  [unwired: 1 in, 1 out]
          }
          frame True {
            n195 = disable-structure shown="Enabled" {
              disable-tunnel: w406 -> [w407 _]
              frame Enabled {
                n196 = local write "TemplateROI"(w407) -> ()
              }
              frame Disabled {
              }
            }
          }
        }
      }
      frame "ClearOverlay" {
        n197 = local read "Vision_Image"() -> (w412:T3)
        n198 = call "IMAQ Clear Overlay"("Image"=w412) -> ("Image Out"=w411:T3)  [unwired: 9 in, 1 out]
        n199 = local write "Vision_Image"(w411) -> ()
      }
      frame "Load Template" {
        # "這個不需要改，因為這是開放給使用者自己去選的"
        # "後面不需要去做Learn Pattern的動作，因為讀進的Pattern都是已經Learn過"
        n200 = Build Path(base path=w421, name or relative path="\\Data") -> (appended path=w420:path)
        n201 = call "File Dialog"("start path"=w420) -> ("selected path"=w419:path, "cancelled"=w418:bool, "error out"=w417:errorcluster)  [unwired: 11 in, 1 out]
        n202 = call <vilib>:"Clear Errors.vi"("error in (no error)"=w417) -> ()  [unwired: 5 in, 2 out]
        n203 = case shown="False" w418 {
          tunnel: w422 -> [w428 w429]
          tunnel: [w427 w429] -> w414
          tunnel: w419 -> [w426 _]
          frame False {
            n204 = call "PatternMatch_ReadTemplate.vi"("template path"=w426, "Template"=w428) -> ("Template Out"=w427:T3)  [unwired: 8 in, 1 out]
          }
          frame True {
          }
        }
        n205 = local write "Template Image"(w414) -> ()
        n206 = call "IMAQ ImageToArray"("Image"=w414) -> ("Image Pixels (U8)"=w415:u8[][])  [unwired: 3 in, 4 out]
        n207 = Empty Array?(array=w415) -> (empty?=w413:bool)
        n208 = case shown="False" w413 {
          frame False {
            n209 = property on="Done" class="Bool"("DisabledEnum"=T12."Enabled" ("Disabled")) -> ()  [unwired: 2 in, 2 out]
          }
          frame True {
          }
        }
      }
    }
    n210 = call <vilib>:"Clear Errors.vi"("error in (no error)"=w56) -> ("error out"=w57:errorcluster)  [unwired: 5 in, 1 out]
  }
  "error out" <- w3
  "Cancel?" <- w38
  n211 = while {
    tunnel: w27 -> [w433]
    tunnel: w15 -> [w432]
    tunnel: w20 -> [w431]
    tunnel: [w430] -> w17
    stop <- w434 stop-if-true
    n212 = event shown="[8] \"Vision_Image\": Mouse Down" {
      selector: w431 -> [_ _ _ _ _ _ _ _ _ _]
      dyn-events: [_ _ _ _ _ _ _ _ _ _] -> w430
      timeout: _ -> [_ _ _ _ _ _ _ _ _ _]
      tunnel: [_ TRUE TRUE TRUE _ _ _ _ _ _] -> w434
      tunnel: w433 -> [_ w438 w442 w446 w454 w459 w471 w473 _ w479]
      tunnel: w432 -> [_ w437 w441 w445 w453 w458 w470 w472 _ w478]
      event Timeout {
        n213 = event-data() -> ()  [unwired: 1 in, 2 out]
      }
      event "Done": Value Change {
        n214 = event-data() -> ()  [unwired: 1 in, 6 out]
        n215 = local read "Match Saturation Threshold 2"() -> (w435:i32)
        n216 = Enqueue Element(queue=w438, element=ColorMatch_UI_Command."Done", error in (no error)=w437) -> ()  [unwired: 1 in, 3 out]
        n217 = local write "Match Saturation Threshold"(w435) -> ()
      }
      event "Cancel": Value Change {
        n218 = event-data() -> ()  [unwired: 1 in, 6 out]
        n219 = Enqueue Element(queue=w442, element=ColorMatch_UI_Command."Cancel", error in (no error)=w441) -> ()  [unwired: 1 in, 3 out]
      }
      event User Event {
        n220 = event-data() -> ()  [unwired: 1 in, 1 out]
        n221 = Enqueue Element(queue=w446, element=ColorMatch_UI_Command."Cancel", error in (no error)=w445) -> ()  [unwired: 1 in, 3 out]
      }
      event "Run Algorithm": Value Change {
        n222 = event-data() -> ()  [unwired: 1 in, 6 out]
        n223 = local read "Match Saturation Threshold 2"() -> (w448:i32)
        n224 = Enqueue Element(queue=w454, element=ColorMatch_UI_Command."RunAlgorithm", error in (no error)=w453) -> (queue out=w450:refnum<queue>, error out=w451:errorcluster)  [unwired: 1 in, 1 out]
        n225 = local write "Match Saturation Threshold"(w448) -> ()
        n226 = Enqueue Element(queue=w450, element=ColorMatch_UI_Command."Draw Overlay", error in (no error)=w451) -> ()  [unwired: 1 in, 3 out]
      }
      event "SetTemplate": Value Change {
        n227 = event-data() -> ()  [unwired: 1 in, 6 out]
        n228 = Enqueue Element(queue=w459, element=ColorMatch_UI_Command."SetTemplate", error in (no error)=w458) -> (queue out=w456:refnum<queue>, error out=w455:errorcluster)  [unwired: 1 in, 1 out]
        n229 = disable-structure shown="Enabled" {
          disable-tunnel: w456 -> [w462 _]
          disable-tunnel: w455 -> [w461 _]
          frame Disabled {
            n230 = Enqueue Element(queue=w462, element=T20."RunAlgorithm", error in (no error)=w461) -> ()  [unwired: 1 in, 3 out]
          }
          frame Enabled {
          }
        }
      }
      event "SetROI": Value Change {
        n231 = event-data() -> ()  [unwired: 1 in, 6 out]
        n232 = Enqueue Element(queue=w471, element=ColorMatch_UI_Command."SetROI", error in (no error)=w470) -> (queue out=w468:refnum<queue>, error out=w467:errorcluster)  [unwired: 1 in, 1 out]
        n233 = Enqueue Element(queue=w468, element=ColorMatch_UI_Command."RunAlgorithm", error in (no error)=w467) -> (queue out=w464:refnum<queue>, error out=w465:errorcluster)  [unwired: 1 in, 1 out]
        n234 = Enqueue Element(queue=w464, element=ColorMatch_UI_Command."Draw Overlay", error in (no error)=w465) -> ()  [unwired: 1 in, 3 out]
      }
      event "Vision_Image": Mouse Up {
        w474 = i32[] [2] items=["No Event"=0, "Click Event"=1, "Draw Event"=2, "Size Event"=4, "Scroll Event"=5, "Double Click Event"=8] ("Which Events")
        n235 = event-data() -> ()  [unwired: 1 in, 8 out]
        n236 = invoke on="Vision_Image" class="ImageControl" method="Get Last Event"("Which Events"=w474) -> ("Type"=w475:i32)  [unwired: 7 in, 7 out]
        n237 = Not Equal To 0?(x=w475) -> (x != 0?=w476:bool)
        n238 = case shown="False" w476 {
          tunnel: w473 -> [_ _]
          tunnel: w472 -> [_ _]
          frame False {
          }
          frame True {
          }
        }
      }
      event "Vision_Image": Mouse Down {
        n239 = event-data() -> ()  [unwired: 1 in, 8 out]
      }
      event Menu Selection (User) {
        n240 = event-data() -> ()  [unwired: 1 in, 8 out]
        n241 = Enqueue Element(queue=w479, element=ColorMatch_UI_Command."Load Template", error in (no error)=w478) -> ()  [unwired: 1 in, 3 out]
      }
    }
  }
  n242 = Unregister For Events(event registration refnum=w17) -> ()  [unwired: 1 in, 1 out]
  n243 = disable-structure shown="Disabled" {
    disable-tunnel: w39 -> [w480 _]
    frame Disabled {
      n244 = call "IMAQ Dispose"("Image"=w480) -> ("error out"=w481:errorcluster)  [unwired: 5 in]
      n245 = call <vilib>:"General Error Handler.vi"("error in (no error)"=w481) -> ()  [unwired: 2 in, 13 out]
    }
    frame Enabled {
    }
  }
  n246 = Destroy User Event(user event=w18) -> (error out=w14:errorcluster)  [unwired: 1 in]
  n247 = call "IMAQ Dispose"("Image"="ColorMatch Image" ("Image Name"), "error in (no error)"=w14) -> ("error out"=w12:errorcluster)  [unwired: 4 in]
  n248 = Flush Queue(queue=w26) -> (queue out=w29:refnum<queue>, error out=w28:errorcluster)  [unwired: 1 in, 1 out]
  n249 = call "IMAQ Dispose"("Image"="ColorMatch Template" ("Image Name"), "error in (no error)"=w12) -> ()  [unwired: 4 in, 1 out]
  n250 = Release Queue(queue=w29, error in (no error)=w28) -> ()  [unwired: 1 in, 3 out]
